vi "StopRecive.vi"(8 "error in (no error)":errorcluster caption="Fehler (Eingang, kein Fehler)", 11 "MoveoSerial Eingang":refnum<class "MoveoSerial.lvclass">) -> (0 "error out":errorcluster caption="Fehler (Ausgang)", 3 "MoveoSerial Ausgang":refnum<class "MoveoSerial.lvclass">)   [LabVIEW 2019, in "MoveoSerial.lvclass"]
uses:
  MoveoSerial.lvclass
  MoveoSerial.lvclass/MoveoSerial.ctl
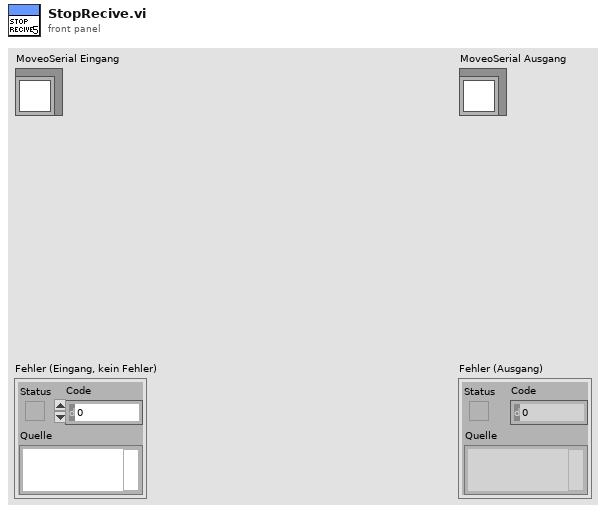
[diagram p1: front panel]
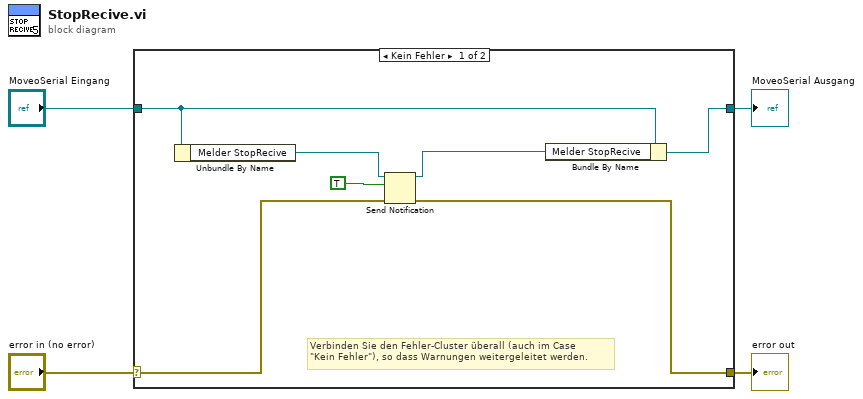
[diagram p0: block diagram]
diagram:
  n1 = case shown="Kein Fehler" "error in (no error)" {
    selector: "error in (no error)" -> [w7 w13]
    tunnel: [w6 w13] -> w3
    tunnel: [w10 w12] -> w1
    tunnel: "MoveoSerial Eingang" -> [w11 w12]
    frame No Error {
      # "Verbinden Sie den Fehler-Cluster überall (auch im Case\n\"Kein Fehler\"), so dass Warnungen weitergeleitet werden."
      n2 = Unbundle By Name(w11) -> ("Melder StopRecive"=w9:refnum<notifier>)
      n3 = Send Notification(notification=TRUE ("Meldung"), notifier=w9, error in (no error)=w7) -> (notifier out=w8:refnum<notifier>, error out=w6:errorcluster)
      n4 = Bundle By Name(cluster=w11, "Melder StopRecive"=w8) -> (w10:refnum<class "MoveoSerial.lvclass">)
    }
    frame Error {
    }
  }
  "error out" <- w3
  "MoveoSerial Ausgang" <- w1
